vi "FichierExisteEtEstTermine.vi"(0 "cheminProchainFichierRAW":path, 2 "entrée d'erreur (pas d'erreur)":errorcluster) -> (3 "path out":path, 4 "ExisteEtTermine":bool, 5 "nomFichier":string, 6 "sortie d'erreur":errorcluster)   [LabVIEW 2017]
panel:
  out "size (in bytes)":i64
  out "file or folder exists?":bool caption="le fichier ou dossier existe ?"
  out "taille":i64
  out "Commande numérique":i32
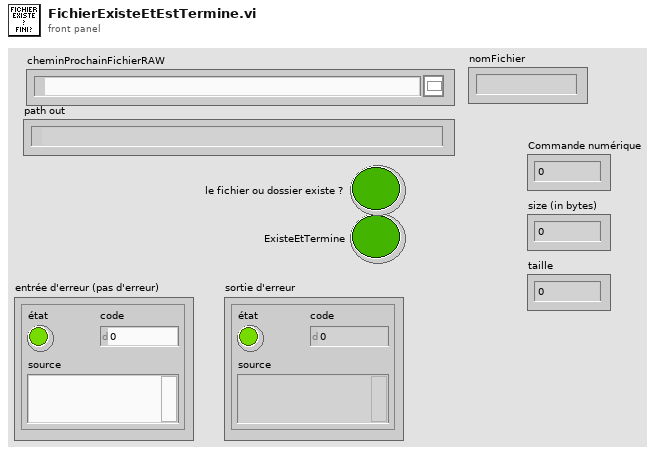
[diagram p1: front panel]
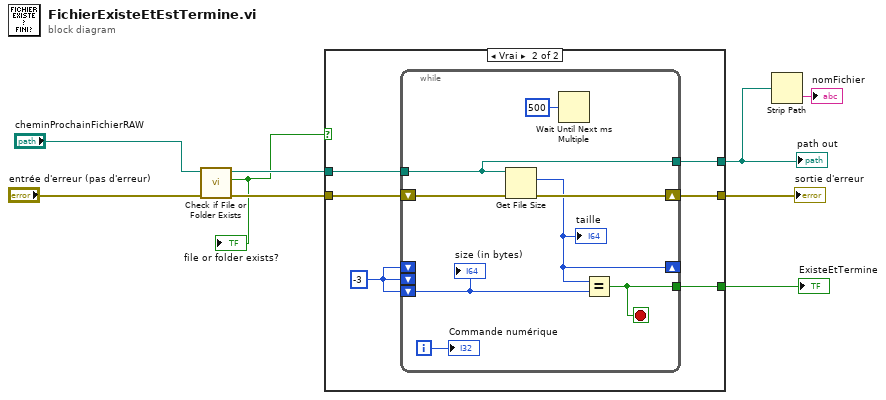
[diagram p0: block diagram]
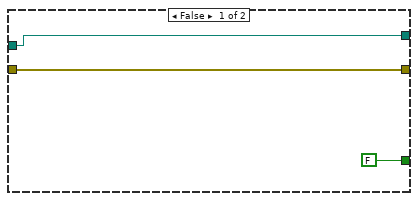
[diagram p2: hidden frame]
diagram:
  n1 = call <vilib>:"Check if File or Folder Exists.vi"("error in (no error)"="entrée d'erreur (pas d'erreur)", "path"="cheminProchainFichierRAW") -> ("error out"=w7:errorcluster, "file or folder exists?"=w4:bool, "dup path"=w9:path)  [unwired: 7 in]
  "file or folder exists?" <- w4
  n2 = case shown="Vrai" w4 {
    tunnel: [w11 w15] -> w2
    tunnel: w9 -> [w11 w16]
    tunnel: [w10 w18] -> w8
    tunnel: w7 -> [w10 w17]
    tunnel: [FALSE w13] -> w3
    frame False {
    }
    frame True {
      w14 = i64 -3 ("size (in bytes)")
      n3 = while {
        shift-right: [w23] -> w18
        shift-left: w17 -> [w24]
        shift-right: [w21] -> _
        shift-left: w14 -> [_]
        tunnel: w16 -> [w22]
        tunnel: [w22] -> w15
        shift-left: w14 -> [_]
        shift-left: w14 -> [w20]
        tunnel: [w19] -> w13
        i -> [w26]
        stop <- w19 stop-if-true
        n4 = Get File Size(file=w22, error in=w24) -> (size (in bytes)=w21:i64, 0:w23:errorcluster)  [unwired: 1 out]
        "taille" <- w21
        n5 = Wait Until Next ms Multiple(millisecond multiple=u32 500 ("n millisecondes")) -> ()  [unwired: 1 out]
        n6 = Equal?(x=w21, y=w20) -> (x = y?=w19:bool)
        "Commande numérique" <- w26
        "size (in bytes)" <- w20
      }
    }
  }
  "path out" <- w2
  "ExisteEtTermine" <- w3
  "sortie d'erreur" <- w8
  n7 = Strip Path(path=w2) -> (name=→"nomFichier":string)  [unwired: 1 out]
